vi "Position_Micos.vi"() -> ()   [LabVIEW 2013, in "Micos_uic.lvlib"]
uses:
  <instrlib>/Micos_uic/Micos_uic.lvlib
panel:
  in  "tickcount_pos":u32
  out "Moving(Micos)":bool
  in  "Position(Micos)":dbl[](array[numeric]) caption="Position" format="%.4f"
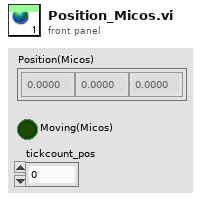
[diagram p1: front panel]
diagram:
